vi "InfoStep.vi"(8 "error in":errorcluster, 10 "Seleziona Step":i32, 11 "Test Steps List":T1[](array[typedef])) -> (0 "error out":errorcluster, 3 "Info Test":string)   [LabVIEW 2019]
doc: "Formatta le informazioni principali degli step in una info box più leggibile"
uses:
  ByteGSAPIBase/TypeDef/Step.ctl
  ByteGSAPIBase/TypeDef/Asset.ctl
  ByteGSAPIBase/ByteGSAPIBase.lvclass
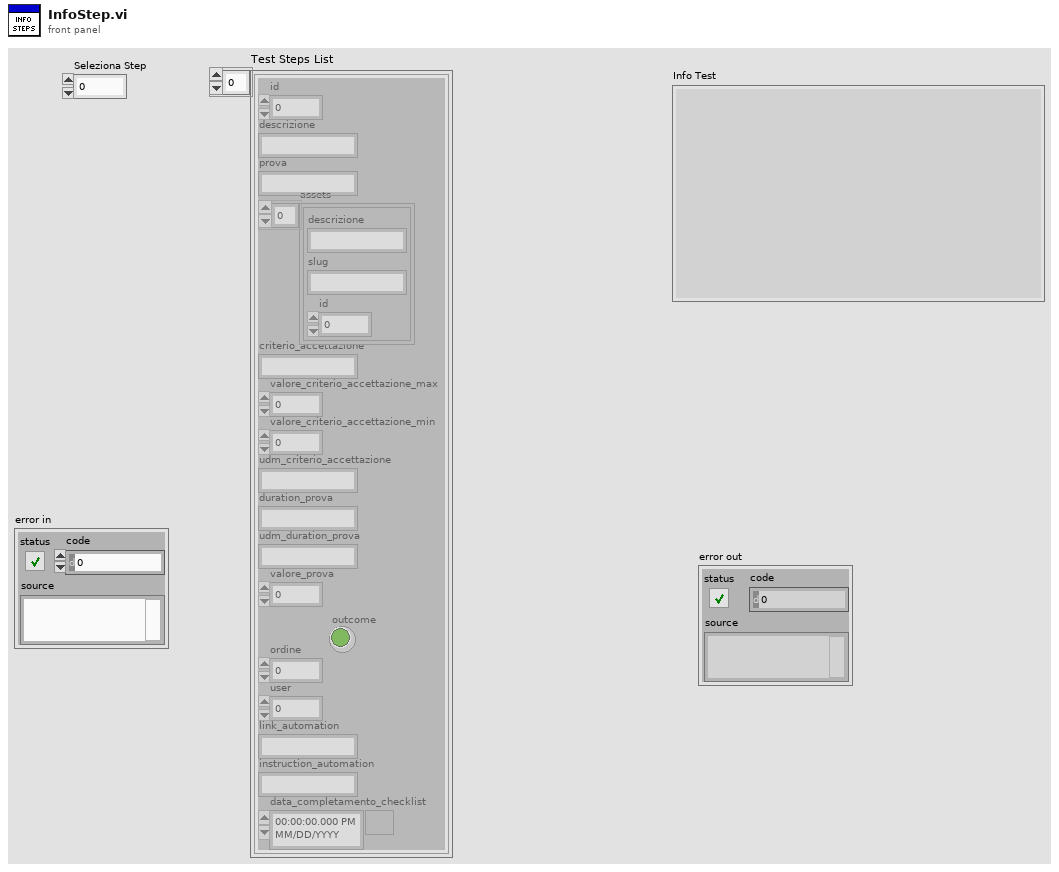
[diagram p1: front panel]
types:
  T1 = typedef "ByteGSWebAPI.lvlib/ByteGSAPIBase.lvclass/Step.ctl" = cluster{"id":i32, "descrizione":string, "prova":string, "assets":T2[], "criterio_accettazione":string, "valore_criterio_accettazione_max":dbl, "valore_criterio_accettazione_min":dbl, "udm_criterio_accettazione":string, "duration_prova":string, "udm_duration_prova":string, "valore_prova":dbl, "ordine":i32, "user":i32, "link_automation":string, "instruction_automation":string, "data_completamento_checklist":timestamp, "outcome":bool}
  T2 = typedef "ByteGSWebAPI.lvlib/ByteGSAPIBase.lvclass/Asset.ctl" = cluster{"descrizione":string, "slug":string, "id":i32}
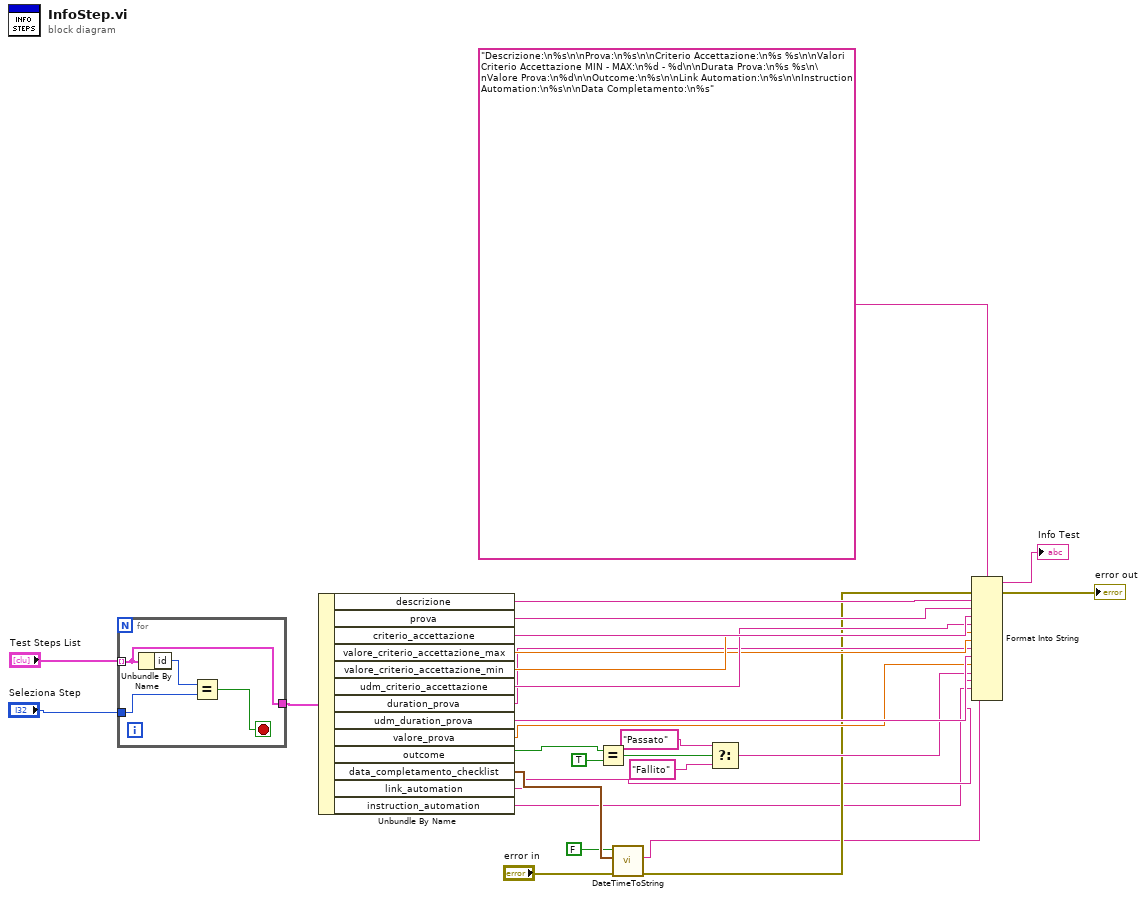
[diagram p0: block diagram]
diagram:
  n1 = for {
    tunnel: "Test Steps List" -> [w29] mode=indexing
    tunnel: "Seleziona Step" -> [w32]
    tunnel: [w29] -> w28
    stop <- w30 stop-if-true
    n2 = Unbundle By Name(w29) -> ("id"=w31:i32)
    n3 = Equal?(x=w31, y=w32) -> (x = y?=w30:bool)
  }
  n4 = Unbundle By Name(w28) -> ("descrizione"=w18:string, "prova"=w17:string, "criterio_accettazione"=w16:string, "valore_criterio_accettazione_max"=w13:dbl, "valore_criterio_accettazione_min"=w14:dbl, "udm_criterio_accettazione"=w15:string, "duration_prova"=w12:string, "udm_duration_prova"=w11:string, "valore_prova"=w10:dbl, "outcome"=w20:bool, "data_completamento_checklist"=w25:timestamp, "link_automation"=w4:string, "instruction_automation"=w3:string)
  n5 = Equal?(x=w20, y=TRUE) -> (x = y?=w22:bool)
  n6 = call "DateTimeToString.vi"("error in"="error in", "current time"=w25, "include Time?"=FALSE ("Time")) -> ("error out"=w7:errorcluster, "Date string"=w2:string)  [unwired: 7 in]
  n7 = Select(t="Passato" ("y"), s=w22, f="Fallito" ("y")) -> (s? t:f=w9:string)
  n8 = Format Into String(format string="Descrizione:\n%s\n\nProva:\n%s\n\nCriterio Accettazione:\n%s %s\n\nValori Criterio Accettazione MIN - MAX:\n%d - %d\n\nDurata Prova:\n%s %s\n\nValore Prova:\n%d\n\nOutcome:\n%s\n\nLink Automation:\n%s\n\nInstruction Automation:\n%s\n\nData Completamento:\n%s", error in=w7, w18, w17, w16, w15, w14, w13, w12, w11, w10, w9, w4, w3, w2) -> (resulting string=→"Info Test":string, error out=→"error out":errorcluster)  [unwired: 1 in]
